vi "RampRateSingle.vi"(6 "return immediately":bool, 7 "ramp rate":dbl, 8 "error in (no error)":T1, 9 "task id":i32(ring) items=["TLibrary", "T01", "T02", "T03", "T04", "T05", "T06", "T07", "T08", "T09", "T10", "T11", "T12", "T13", "T14", "T15", "T16", "T17", "T18", "T19", "T20", "T21", "T22", "T23", "T24", "T25", "T26", "T27", "T28", "T29", "T30", "T31"], 10 "axis name":string, 11 "controller in":refnum<k24>) -> (0 "error out (no error)":T1, 3 "controller out":refnum<k24>)   [LabVIEW 2010]
doc: "Acceleration and Deceleration rates are set to ramp rate for the specified axis."
uses:
  c:/aerotech/controller/stable/A3200/pc/labview/2010/bin/Aerotech.A3200.dll
  bin/Aerotech.A3200.dll
  c:/aerotech/controller/stable/A3200/pc/labview/2010/bin/Aerotech.A3200.LabVIEW.dll
  bin/Aerotech.A3200.LabVIEW.dll
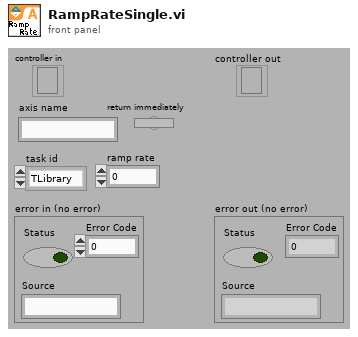
[diagram p1: front panel]
types:
  T1 = cluster{"Status":bool, "Error Code":i32, "Source":string}
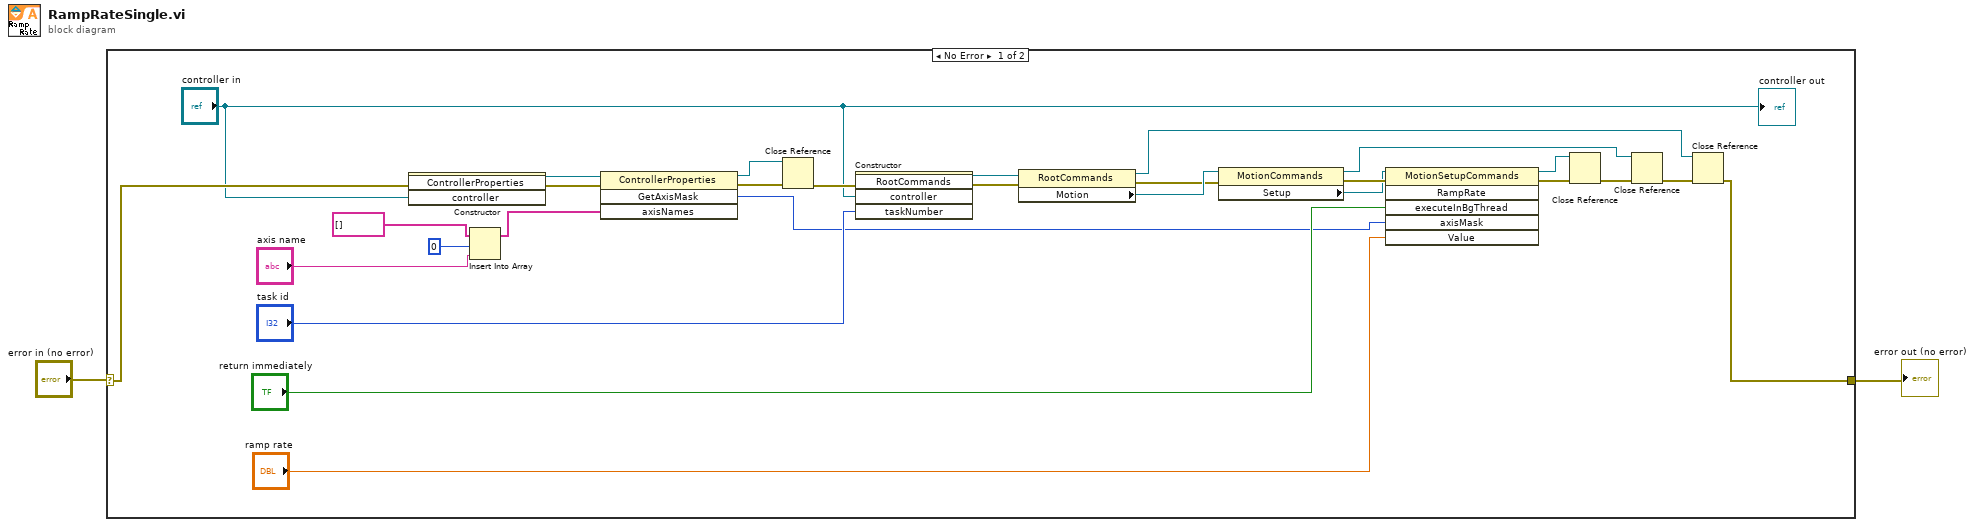
[diagram p0: block diagram]
diagram:
  n1 = case shown="No Error" "error in (no error)" {
    selector: "error in (no error)" -> [w25 w31]
    tunnel: [w8 w31] -> w1
    frame No Error {
      n2 = constructor class="ControllerProperties"(error in=w25, "controller"="controller in") -> (reference out=w30:refnum<k24>, error out=w29:errorcluster)  [unwired: 2 in, 2 out]
      n3 = Insert Into Array(array=string[] [], index=0, new element="axis name") -> (w3:string[])
      n4 = invoke class="ControllerProperties" method="GetAxisMask"(reference=w30, error in=w29, "axisNames"=w3) -> (reference out=w27:refnum<k24>, error out=w28:errorcluster, "GetAxisMask"=w15:i32)  [unwired: 1 in, 1 out]
      n5 = Close Reference(reference=w27, error in (no error)=w28) -> (error out=w26:errorcluster)
      n6 = constructor class="RootCommands"(error in=w26, "controller"="controller in", "taskNumber"="task id") -> (reference out=w22:refnum<k24>, error out=w23:errorcluster)  [unwired: 2 in, 3 out]
      n7 = property class="RootCommands"(reference=w22, error in=w23) -> (reference out=w9:refnum<k24>, error out=w20:errorcluster, "Motion"=w21:refnum<k24>)
      n8 = property class="MotionCommands"(reference=w21, error in=w20) -> (reference out=w10:refnum<k24>, error out=w19:errorcluster, "Setup"=w18:refnum<k24>)
      n9 = invoke class="MotionSetupCommands" method="RampRate"(reference=w18, error in=w19, "executeInBgThread"="return immediately", "axisMask"=w15, "Value"="ramp rate") -> (reference out=w13:refnum<k24>, error out=w14:errorcluster)  [unwired: 1 in, 4 out]
      n10 = Close Reference(reference=w13, error in (no error)=w14) -> (error out=w12:errorcluster)
      n11 = Close Reference(reference=w10, error in (no error)=w12) -> (error out=w11:errorcluster)
      n12 = Close Reference(reference=w9, error in (no error)=w11) -> (error out=w8:errorcluster)
      "controller out" <- "controller in"
    }
    frame Error {
    }
  }
  "error out (no error)" <- w1
